vi "picoquant_process_loop.vi"(8 "error in (no error)":errorcluster, 10 "ui_user_events":T1, 11 "picoquant_generic in":refnum<class "picoquant_generic.lvclass">) -> (0 "error out":errorcluster, 3 "picoquant_generic out":refnum<class "picoquant_generic.lvclass">)   [LabVIEW 2015, in "picoquant_generic.lvclass"]
uses:
  picoquant_generic.lvclass
  UI/front_panel_class/ui_user_events.ctl
  picoquant_generic.lvclass/picoquant_generic.ctl
  loop_notifier_tdef.ctl
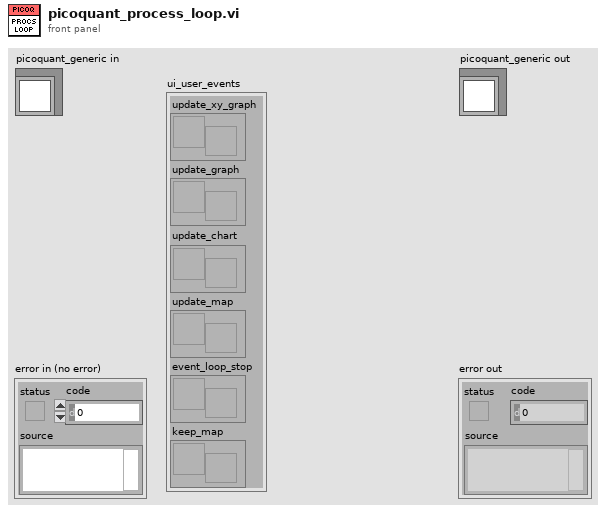
[diagram p1: front panel]
types:
  T1 = typedef "ui_user_events.ctl" = cluster{"update_xy_graph":refnum<user-event>, "update_graph":refnum<user-event>, "update_chart":refnum<user-event>, "update_map":refnum<user-event>, "event_loop_stop":refnum<user-event>, "keep_map":refnum<user-event>}
  T2 = typedef "loop_notifier_tdef.ctl" = enum16{"exit"}
  T3 = typedef "picoquant_data_tdef.ctl" = cluster{"channels":u8[], "times":u64[], "sync":u64[]}
  T4 = typedef "processing_tasks_tdef.ctl" = enum16{"none", "correlate", "histogram"}
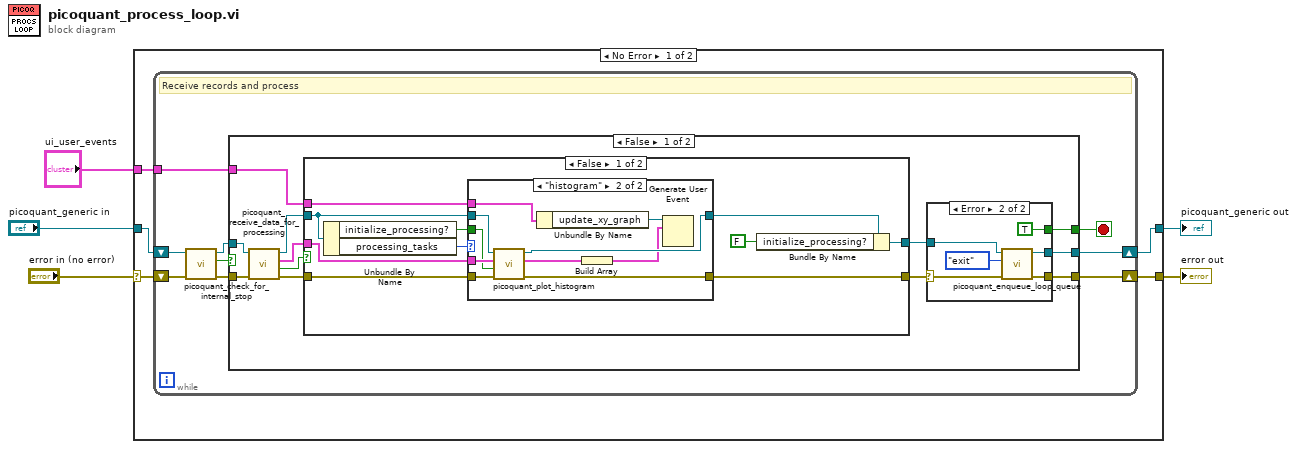
[diagram p0: block diagram]
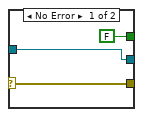
[diagram p4: hidden frame]
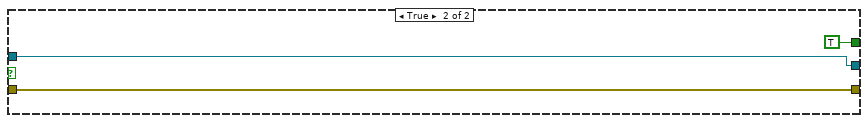
[diagram p5: hidden frame]
diagram:
  n1 = case shown="No Error" "error in (no error)" {
    selector: "error in (no error)" -> [w10 w69]
    tunnel: [w7 w69] -> w4
    tunnel: [w8 w68] -> w2
    tunnel: "picoquant_generic in" -> [w9 w68]
    tunnel: "ui_user_events" -> [w6 _]
    frame No Error {
      n2 = while {
        shift-right: [w14] -> w8
        shift-left: w9 -> [w18]
        shift-right: [w13] -> w7
        shift-left: w10 -> [w19]
        tunnel: w6 -> [w11]
        stop <- w12 stop-if-true
        # "Receive records and process"
        n3 = call "picoquant_check_for_internal_stop.vi"("error in (no error)"=w19, "picoquant_generic in"=w18) -> ("error out"=w16:errorcluster, "exit?"=w17:bool, "picoquant_generic out"=w15:refnum<class "picoquant_generic.lvclass">)  [unwired: 7 in]
        n4 = case shown="False" w17 {
          tunnel: w16 -> [w28 w66]
          tunnel: w15 -> [w27 w67]
          tunnel: [w29 w67] -> w14
          tunnel: [w31 w66] -> w13
          tunnel: [w30 TRUE] -> w12
          tunnel: w11 -> [w20 _]
          frame False {
            n5 = call "picoquant_receive_data_for_processing.vi"("error in (no error)"=w28, "picoquant_generic in"=w27) -> ("error out"=w23:errorcluster, "timed out?"=w26:bool, "data_out"=w21:T3, "picoquant_generic out"=w25:refnum<class "picoquant_generic.lvclass">)  [unwired: 6 in]
            n6 = case shown="False" w26 {
              tunnel: w25 -> [w38 w55]
              tunnel: [w33 w55] -> w24
              tunnel: w23 -> [w39 w54]
              tunnel: [w37 w54] -> w22
              tunnel: w21 -> [w40 _]
              tunnel: w20 -> [w32 _]
              frame False {
                n7 = Unbundle By Name(w38) -> ("initialize_processing?"=w36:bool, "processing_tasks"=w41:T4)
                n8 = case shown="\"histogram\"" w41 {
                  tunnel: w40 -> [_ w53]
                  tunnel: w39 -> [w43 w52]
                  tunnel: w38 -> [w42 w51]
                  tunnel: [w42 w50] -> w35
                  tunnel: [w43 w49] -> w37
                  tunnel: w36 -> [_ w48]
                  tunnel: w32 -> [_ w47]
                  frame "none", Default {
                  }
                  frame "histogram" {
                    n9 = call-dynamic "picoquant_plot_histogram.vi"("error in (no error)"=w52, "initialize_histogram?"=w48, "data"=w53, "picoquant_generic in"=w51) -> ("error out"=w49:errorcluster, "histogram"=w45:cluster{"Axis":dbl[], "Histogram":i32[]}, "picoquant_generic out"=w50:refnum<class "picoquant_generic.lvclass">)  [unwired: 5 in]
                    n10 = Unbundle By Name(w47) -> ("update_xy_graph"=w46:refnum<user-event>)
                    n11 = Build Array(w45) -> (w44:cluster{"Axis":dbl[], "Histogram":i32[]}[])
                    n12 = Generate User Event(user event=w46, event data cluster=w44) -> ()  [unwired: 2 in, 2 out]
                  }
                }
                n13 = Bundle By Name(cluster=w35, "initialize_processing?"=FALSE) -> (w33:refnum<class "picoquant_generic.lvclass">)
              }
              frame True {
              }
            }
            n14 = case shown="Error" w22 {
              selector: w22 -> [w58 w62]
              tunnel: w24 -> [w56 w64]
              tunnel: [w58 w59] -> w31
              tunnel: [FALSE TRUE] -> w30
              tunnel: [w56 w60] -> w29
              frame No Error {
              }
              frame Error {
                n15 = call "picoquant_enqueue_loop_queue.vi"("error in (no error)"=w62, "loop_notifier"=loop_notifier_tdef."exit" ("element"), "picoquant_generic in"=w64) -> ("error out"=w59:errorcluster, "picoquant_generic out"=w60:refnum<class "picoquant_generic.lvclass">)  [unwired: 7 in]
              }
            }
          }
          frame True {
          }
        }
      }
    }
    frame Error {
    }
  }
  "error out" <- w4
  "picoquant_generic out" <- w2
